vi "Number_2_string.vi"(1 "precision":string, 2 "number":dbl format="%.5f") -> (0 "String":string)   [LabVIEW 2010]
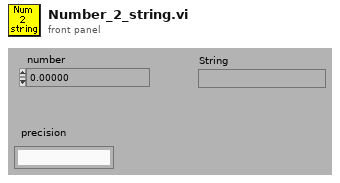
[diagram p1: front panel]
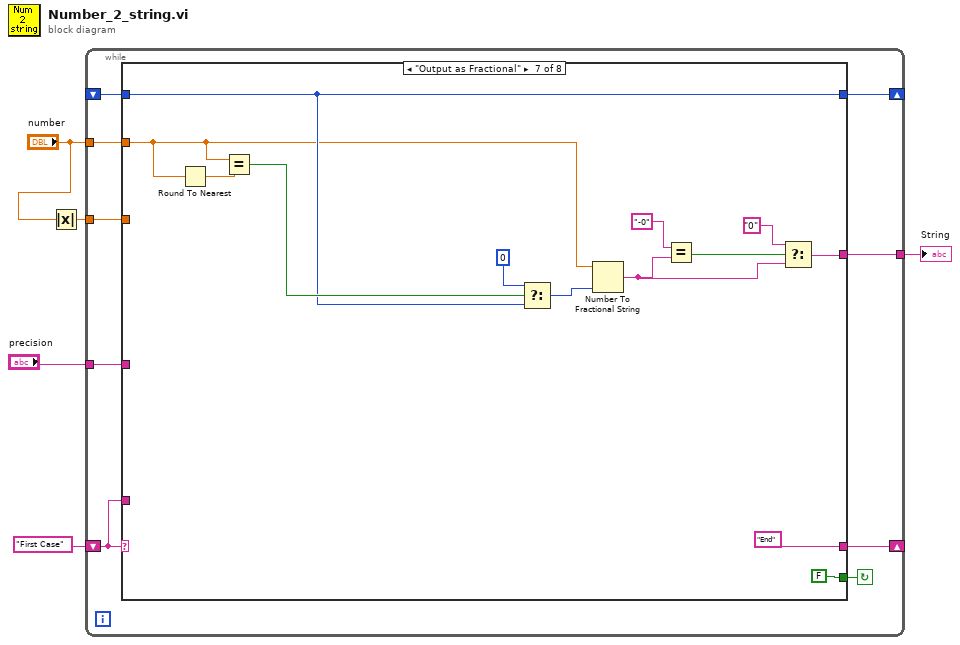
[diagram p0: block diagram]
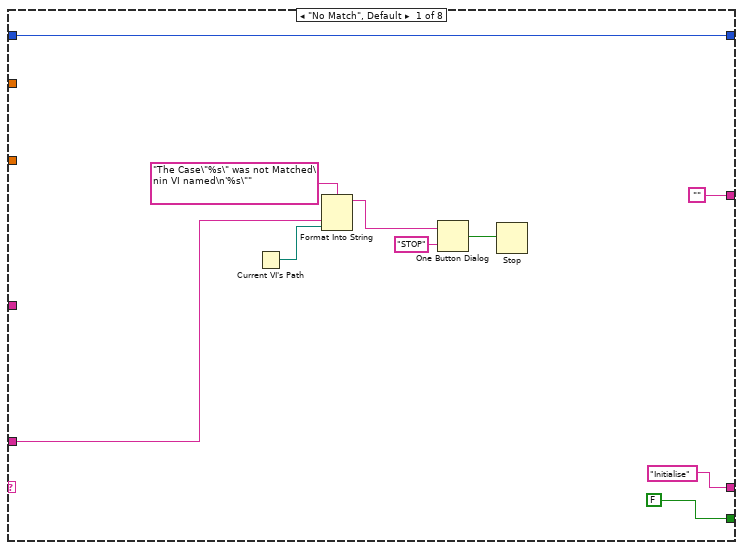
[diagram p2: hidden frame]
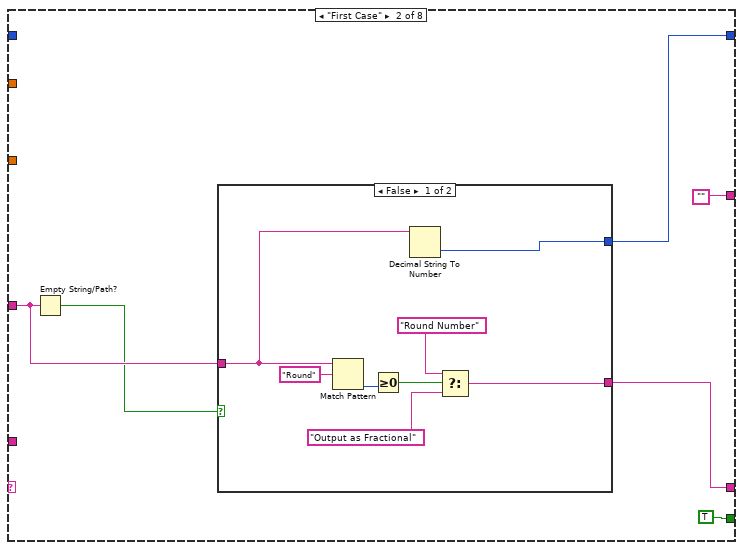
[diagram p3: hidden frame]
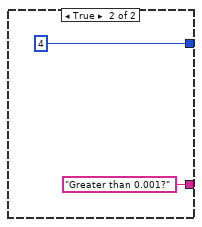
[diagram p4: hidden frame]
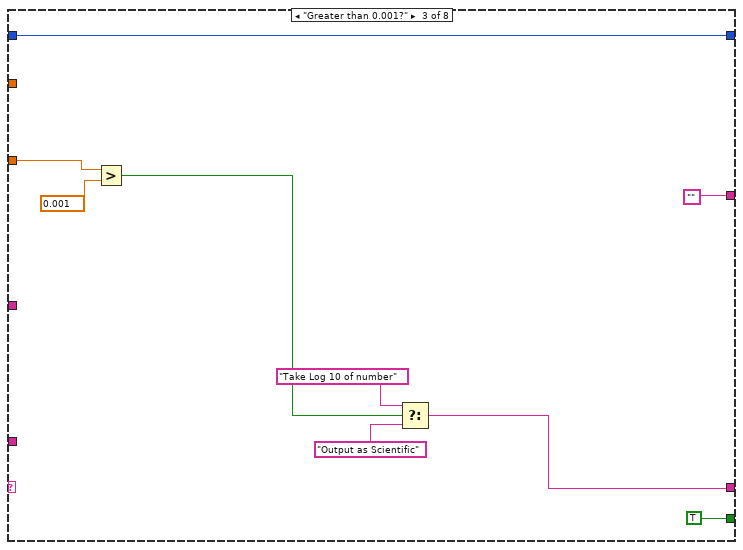
[diagram p5: hidden frame]
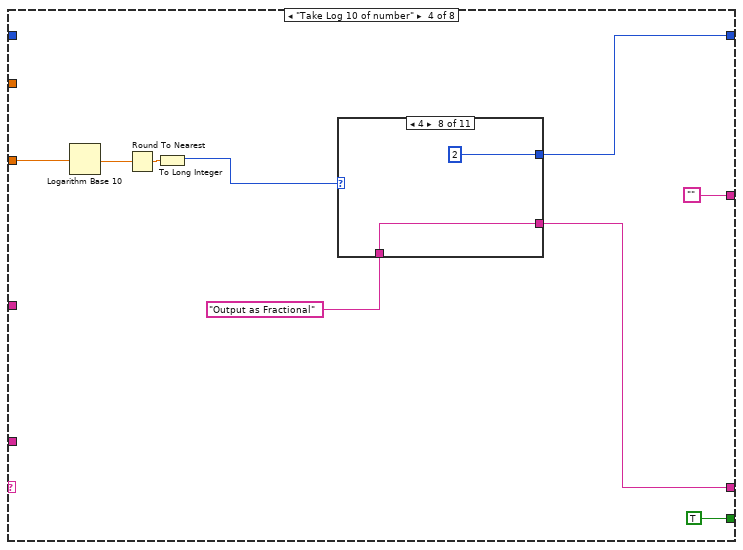
[diagram p6: hidden frame]
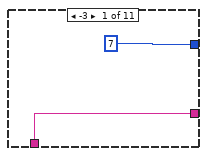
[diagram p7: hidden frame]
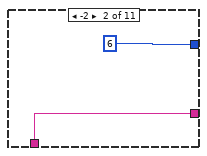
[diagram p8: hidden frame]
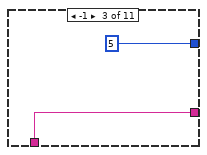
[diagram p9: hidden frame]
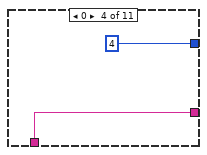
[diagram p10: hidden frame]
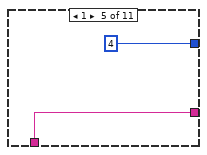
[diagram p11: hidden frame]
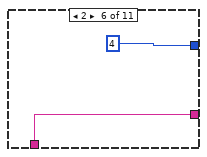
[diagram p12: hidden frame]
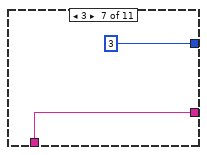
[diagram p13: hidden frame]
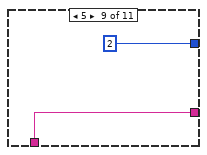
[diagram p14: hidden frame]
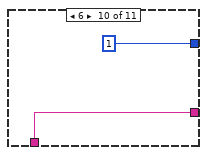
[diagram p15: hidden frame]
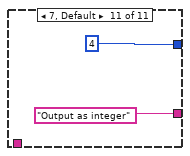
[diagram p16: hidden frame]
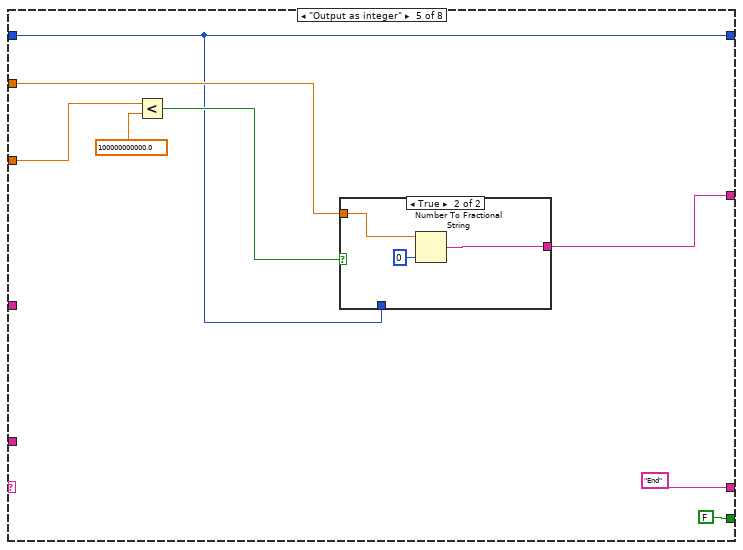
[diagram p17: hidden frame]
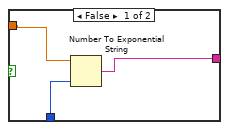
[diagram p18: hidden frame]
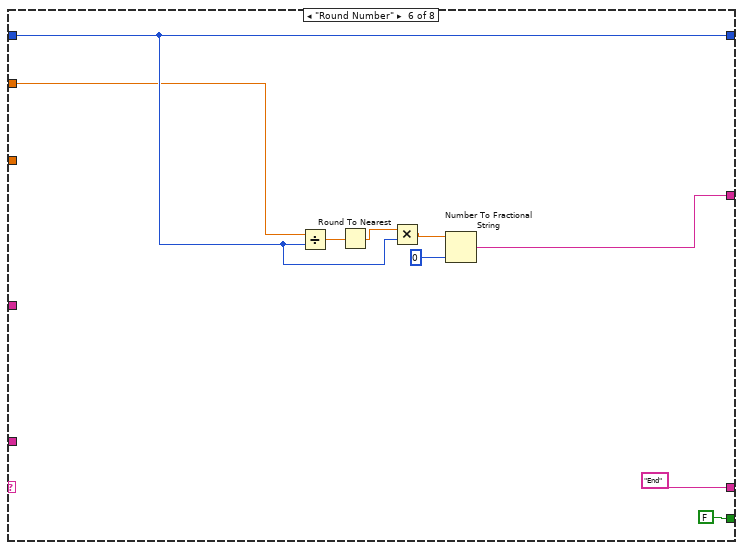
[diagram p19: hidden frame]
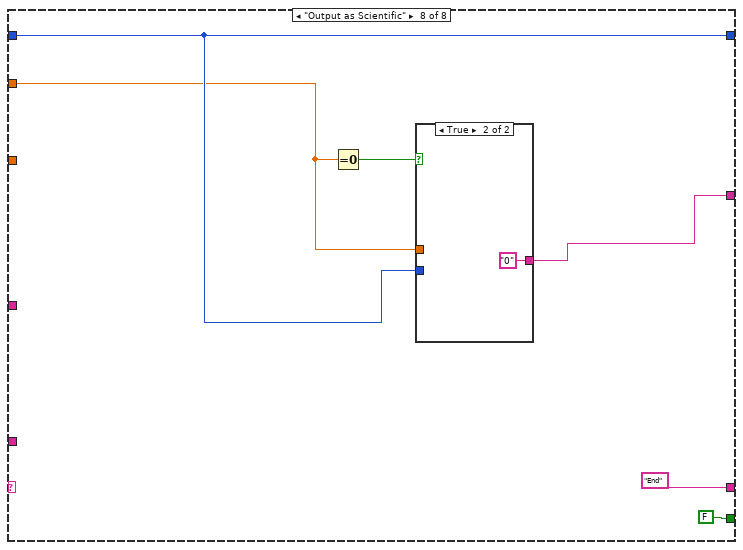
[diagram p20: hidden frame]
diagram:
  n1 = Absolute Value(x="number") -> (abs(x)=w2:dbl)
  n2 = while {
    shift-left: "First Case" -> [w12]
    shift-right: [w13] -> _
    tunnel: "precision" -> [w11]
    tunnel: "number" -> [w10]
    tunnel: w2 -> [w9]
    tunnel: [w8] -> w1
    shift-right: [w7] -> _
    shift-left: _ -> [w6]
    stop <- w14 continue-if-true
    n3 = case shown="\"Output as Fractional\"" w12 {
      tunnel: [FALSE TRUE TRUE TRUE FALSE FALSE FALSE FALSE] -> w14
      tunnel: ["Initialise" w26 w45 w50 "End" "End" "End" "End"] -> w13
      tunnel: w12 -> [w19 _ _ _ _ _ _ _]
      tunnel: w11 -> [_ w29 _ _ _ _ _ _]
      tunnel: w10 -> [_ _ _ _ w83 w95 w109 w118]
      tunnel: w9 -> [_ _ w47 w57 w85 _ _ _]
      tunnel: ["" "" "" "" w82 w96 w104 w120] -> w8
      tunnel: [w15 w27 w41 w53 w81 w99 w111 w119] -> w7
      tunnel: w6 -> [w15 _ w41 _ w81 w99 w111 w119]
      frame "No Match", Default {
        n4 = Current VI's Path() -> (path=w18:path)
        n5 = Format Into String(format string="The Case\"%s\" was not Matched\nin VI named\n'%s\"" ("Format String"), w19, w18) -> (resulting string=w22:string)  [unwired: 2 in, 1 out]
        n6 = One Button Dialog(message=w22, button name ("OK")="STOP") -> (true=w20:bool)
        n7 = Stop(stop? (T)=w20) -> ()
      }
      frame "First Case" {
        n8 = Empty String/Path?(string/path=w29) -> (empty?=w28:bool)
        n9 = case shown="False" w28 {
          tunnel: w29 -> [w35 _]
          tunnel: [w34 4] -> w27
          tunnel: [w32 "Greater than 0.001?" ("f")] -> w26
          frame False {
            n10 = Match Pattern(string=w35, regular expression="Round") -> (offset past match=w38:i32)  [unwired: 4 out]
            n11 = Greater Or Equal To 0?(x=w38) -> (x >= 0?=w36:bool)
            n12 = Decimal String To Number(string=w35) -> (number=w34:i32)  [unwired: 3 out]
            n13 = Select(t="Round Number", s=w36, f="Output as Fractional") -> (s? t:f=w32:string)
          }
          frame True {
          }
        }
      }
      frame "Greater than 0.001?" {
        n14 = Greater?(x=w47, y=0.001) -> (0:w46:bool)
        n15 = Select(t="Take Log 10 of number", s=w46, f="Output as Scientific") -> (s? t:f=w45:string)
      }
      frame "Take Log 10 of number" {
        n16 = Logarithm Base 10(1:w57) -> (0:w55:dbl)
        n17 = Round To Nearest(number=w55) -> (nearest integer value=w56:dbl)
        n18 = To Long Integer(number=w56) -> (32bit integer=w54:i32)
        n19 = case shown="4" w54 {
          tunnel: [7 6 5 4 4 4 3 2 2 1 4] -> w53
          tunnel: [w59 w61 w63 w65 w67 w69 w71 w73 w75 w77 "Output as integer"] -> w50
          tunnel: "Output as Fractional" -> [w59 w61 w63 w65 w67 w69 w71 w73 w75 w77 _]
          frame -3 {
          }
          frame -2 {
          }
          frame -1 {
          }
          frame 0 {
          }
          frame 1 {
          }
          frame 2 {
          }
          frame 3 {
          }
          frame 4 {
          }
          frame 5 {
          }
          frame 6 {
          }
          frame 7, Default {
          }
        }
      }
      frame "Output as integer" {
        n20 = Less?(x=w85, y=100000000000.0) -> (x < y?=w84:bool)
        n21 = case shown="True" w84 {
          tunnel: [w90 w94] -> w82
          tunnel: w83 -> [w91 w92]
          tunnel: w81 -> [w89 _]
          frame False {
            n22 = Number To Exponential String(number=w91, precision (6)=w89) -> (E-format string=w90:string)  [unwired: 2 out]
          }
          frame True {
            n23 = Number To Fractional String(number=w92, precision (6)=i16 0) -> (F-format string=w94:string)  [unwired: 2 out]
          }
        }
      }
      frame "Round Number" {
        n24 = Divide(x=w95, y=w99) -> (x/y=w101:dbl)
        n25 = Round To Nearest(number=w101) -> (nearest integer value=w100:dbl)
        n26 = Multiply(x=w100, y=w99) -> (x*y=w98:dbl)
        n27 = Number To Fractional String(number=w98, precision (6)=0) -> (F-format string=w96:string)  [unwired: 2 out]
      }
      frame "Output as Fractional" {
        n28 = Round To Nearest(number=w109) -> (nearest integer value=w114:dbl)
        n29 = Equal?(x=w109, y=w114) -> (x = y?=w113:bool)
        n30 = Select(t=0, s=w113, f=w111) -> (s? t:f=w110:i32)
        n31 = Number To Fractional String(number=w109, precision (6)=w110) -> (F-format string=w106:string)  [unwired: 2 out]
        n32 = Equal?(x="-0", y=w106) -> (x = y?=w107:bool)
        n33 = Select(t="0", s=w107, f=w106) -> (s? t:f=w104:string)
      }
      frame "Output as Scientific" {
        n34 = Equal To 0?(x=w118) -> (x = 0?=w117:bool)
        n35 = case shown="True" w117 {
          tunnel: [w125 "0"] -> w120
          tunnel: w119 -> [w124 _]
          tunnel: w118 -> [w123 _]
          frame False {
            n36 = Number To Exponential String(number=w123, precision (6)=w124) -> (E-format string=w125:string)  [unwired: 2 out]
          }
          frame True {
          }
        }
      }
    }
  }
  "String" <- w1
